vi "Begin.vi"(8 "error in":errorcluster) -> (0 "error out":errorcluster)   [LabVIEW 2018]
doc: "Called before other user functions, this VI is expected to open initial I/O refnums, load in file data, and do all program initialization. Notice that the <B>error out</B> terminal is simply used for data flow. Wiring it to other structures or subVIs ensures that this VI runs first."
uses:
  <vilib>/Rock Robotics/WPI/DriverStation/WPI_DriverStationRobotMode2.ctl
  <vilib>/Rock Robotics/WPI/Joystick/WPI_JoystickDeviceEnum.ctl
  <vilib>/Rock Robotics/WPI/ThirdParty/Phoenix-LabVIEW/Motor Controller/Controls/CTRE_Phoenix_MotorControl_ControlMode.ctl
  <vilib>/Rock Robotics/SystemInterfaces/AI/FPGA_AIChannel.ctl
  Robot Global Data.vi
  <vilib>/Rock Robotics/Network Tables/NT Write String Array.vi
panel:
  in  "Do Encoder Reset":bool
  in  "timeoutMs":u32=100
  in  "Back Right Zero":dbl=150.0
  in  "Back Left Zero":dbl=3340.0
  in  "Front Right Zero":dbl=3534.0
  in  "Front Left Zero":dbl=180.0
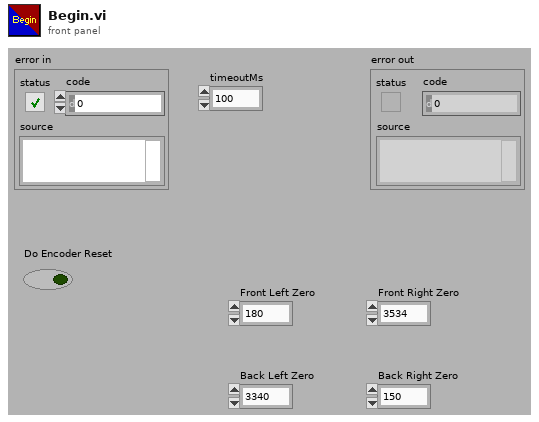
[diagram p1: front panel]
types:
  T1 = typedef "CTRE_Phoenix_MotorControl_ControlMode.ctl" = u16
  T2 = typedef "FPGA_AIChannel.ctl" = enum8{"AI 0", "AI 1", "AI 2", "AI 3", "AI MXP 0", "AI MXP 1", "AI MXP 2", "AI MXP 3", "Invalid"}
  T3 = typedef "WPI_JoystickDeviceEnum.ctl" = enum16{"USB 0", "USB 1", "USB 2", "USB 3", "USB 4", "USB 5"}
  T4 = typedef "WPI_DriverStationRobotMode2.ctl" = enum16{"Autonomous Disabled", "Autonomous Enabled", "Teleop Disabled", "Teleop Enabled", "Disconnected", "Finish", "Test Disabled", "Test Enabled", "Emergency Stopped"}
  T5 = typedef "WPI_MotorControlDeviceRef.ctl" = cluster{"DeviceStatus":errorcluster, "Type":T6, "PWM":cluster{"PWM Channel":T7, "DeadBand":T8}, "CAN":cluster{"Device Number":u8, "SetOutput VI Ref":variant, "GetOutput VI Ref":variant, "Enable VI Ref":variant, "Disable VI Ref":variant, "Data":variant}, "Invert":bool, "DIO PWM":cluster{"PWM \"Enable\" Channel":T7, "DIOChannel":T9, "PWM Rate":dbl}}
  T6 = typedef "WPI_MotorControlType.ctl" = enum16{"PWM", "CAN", "DIO PWM"}
  T7 = typedef "FPGA_DIOPWMChannel.ctl" = enum8{"PWM 0", "PWM 1", "PWM 2", "PWM 3", "PWM 4", "PWM 5", "PWM 6", "PWM 7", "PWM 8", "PWM 9", "PWM MXP 0", "PWM MXP 1", "PWM MXP 2", "PWM MXP 3", "PWM MXP 4", "PWM MXP 5", "PWM MXP 6", "PWM MXP 7", "PWM MXP 8", "PWM MXP 9", "Invalid"}
  T8 = typedef "WPI_PWMDeadband.ctl" = cluster{"Name":string, "maxPositivePwm":i32, "minPositivePwm":i32, "centerPwm":i32, "maxNegativePwm":i32, "minNegativePwm":i32, "angularRange":u16}
  T9 = typedef "FPGA_DIOChannel.ctl" = enum8{"DIO 0", "DIO 1", "DIO 2", "DIO 3", "DIO 4", "DIO 5", "DIO 6", "DIO 7", "DIO 8", "DIO 9", "DIO MXP 0", "DIO MXP 1", "DIO MXP 2", "DIO MXP 3", "DIO MXP 4", "DIO MXP 5", "DIO MXP 6", "DIO MXP 7", "DIO MXP 8", "DIO MXP 9", "DIO MXP 10", "DIO MXP 11", "DIO MXP 12", "DIO MXP 13", "DIO MXP 14", "DIO MXP 15", "SPI Port CS1", "SPI Port CS2", "SPI Port CS3", "SPI Port MISO", "SPI Port MOSI", "Invalid"}
  T10 = typedef "WPI_JoystickDevRef.ctl" = cluster{"Device":T3}
  T11 = typedef "WPI_AnalogChannelDevRef.ctl" = cluster{"DevStatus":errorcluster, "Analog Channel":T2}
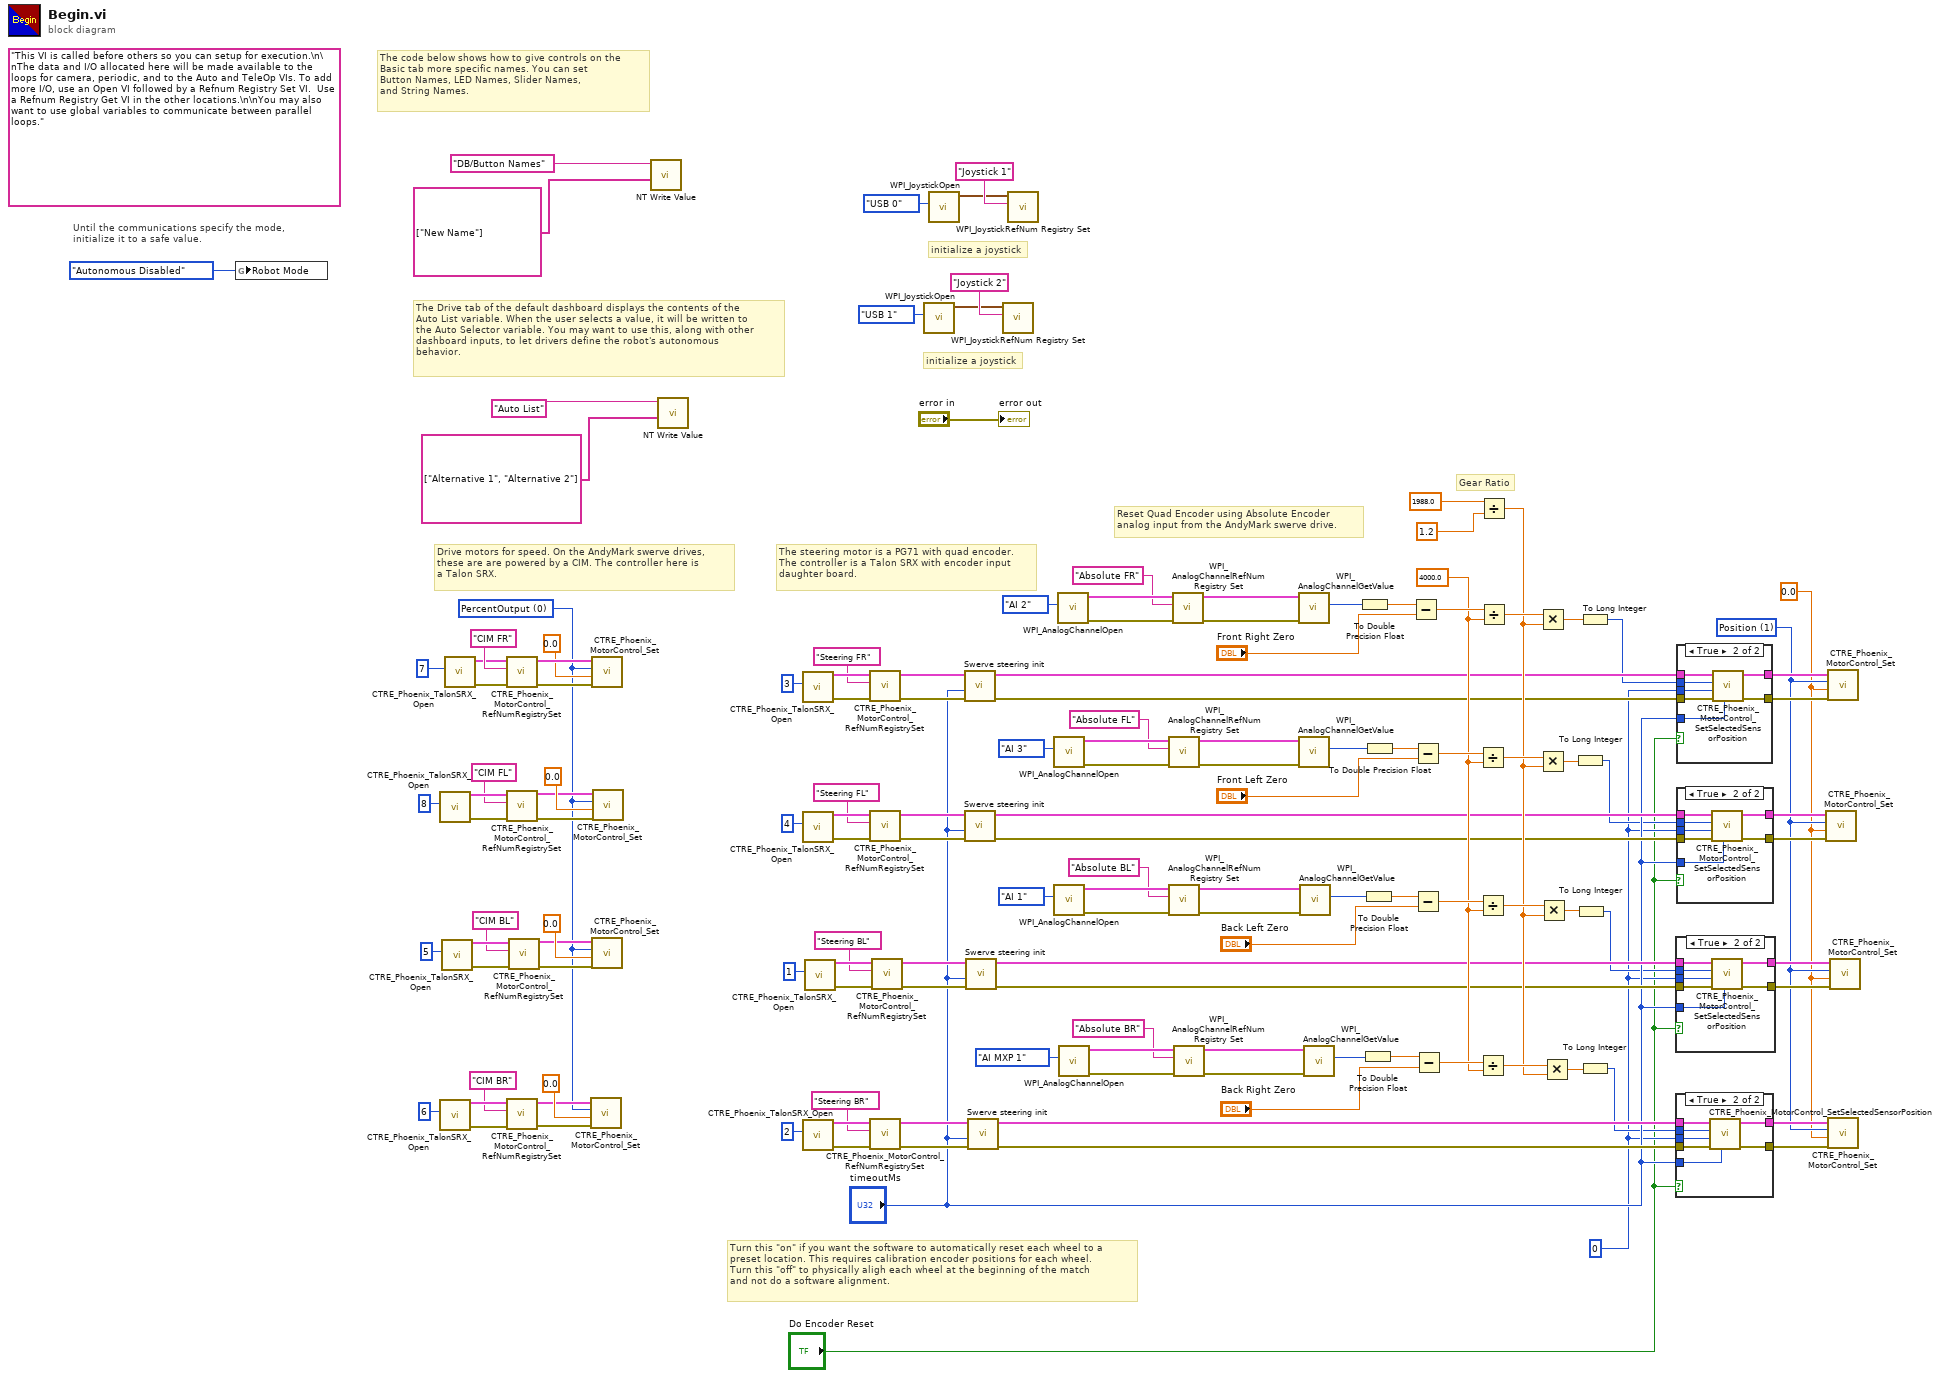
[diagram p0: block diagram]
diagram:
  w10 = 0.0 ("Output")
  w11 = T1 1 items=["PercentOutput"=0, "Position"=1, "Velocity"=2, "Current"=3, "Follower"=5, "MotionProfile"=6, "MotionMagic"=7, "MotionProfileArc"=10, "Disabled"=15] ("Control Mode")
  w20 = u32 0 ("pidLoopIdx")
  w44 = 4000.0 ("x")
  w102 = T1 0 items=["PercentOutput"=0, "Position"=1, "Velocity"=2, "Current"=3, "Follower"=5, "MotionProfile"=6, "MotionMagic"=7, "MotionProfileArc"=10, "Disabled"=15] ("Control Mode")
  (unwired) "This VI is called before others so you can setup for execution.\n\nThe data and I/O allocated here will be made available to the loops for camera, periodic, and to the Auto and TeleOp VIs. To add more I/O, use an Open VI followed by a Refnum Registry Set VI.  Use a Refnum Registry Get VI in the other locations.\n\nYou may also want to use global variables to communicate between parallel loops."
  # "The steering motor is a PG71 with quad encoder.\nThe controller is a Talon SRX with encoder input\ndaughter board."
  # "Drive motors for speed. On the AndyMark swerve drives,\nthese are are powered by a CIM. The controller here is\na Talon SRX."
  # "Turn this \"on\" if you want the software to automatically reset each wheel to a\npreset location. This requires calibration encoder positions for each wheel.\nTurn this \"off\" to physically aligh each wheel at the beginning of the match\nand not do a software alignment."
  # "Gear Ratio"
  # "Reset Quad Encoder using Absolute Encoder\nanalog input from the AndyMark swerve drive."
  # "initialize a joystick"
  # "The Drive tab of the default dashboard displays the contents of the\nAuto List variable. When the user selects a value, it will be written to\nthe Auto Selector variable. You may want to use this, along with other\ndashboard inputs, to let drivers define the robot's autonomous\nbehavior."
  # "The code below shows how to give controls on the\nBasic tab more specific names. You can set\nButton Names, LED Names, Slider Names,\nand String Names."
  # "initialize a joystick"
  # "Until the communications specify the mode,\ninitialize it to a safe value."
  n1 = global write "Robot Global Data.vi" "Robot Mode"(WPI_DriverStationRobotMode2."Autonomous Disabled" ("Robot Mode")) -> ()
  n2 = call <vilib>:"CTRE_Phoenix_TalonSRX_Open.vi"("Device Number"=u8 8) -> ("error out"=w128:errorcluster, "CAN Talon SRX Ref"=w129:T5)  [unwired: 9 in]
  n3 = call <vilib>:"CTRE_Phoenix_TalonSRX_Open.vi"("Device Number"=u8 6) -> ("error out"=w122:errorcluster, "CAN Talon SRX Ref"=w123:T5)  [unwired: 9 in]
  n4 = call <vilib>:"CTRE_Phoenix_TalonSRX_Open.vi"("Device Number"=u8 5) -> ("error out"=w125:errorcluster, "CAN Talon SRX Ref"=w126:T5)  [unwired: 9 in]
  n5 = call <vilib>:"CTRE_Phoenix_TalonSRX_Open.vi"("Device Number"=u8 7) -> ("error out"=w109:errorcluster, "CAN Talon SRX Ref"=w110:T5)  [unwired: 9 in]
  n6 = call <vilib>:"CTRE_Phoenix_MotorControl_RefNumRegistrySet.vi"("error in (no error)"=w109, "refnum name"="CIM FR", "PhoenixMotorControlDevRef"=w110) -> ("error out"=w120:errorcluster, "PhoenixMotorControlDevRef"=w119:T5)  [unwired: 7 in]
  n7 = call <vilib>:"CTRE_Phoenix_MotorControl_RefNumRegistrySet.vi"("error in (no error)"=w128, "refnum name"="CIM FL", "PhoenixMotorControlDevRef"=w129) -> ("error out"=w107:errorcluster, "PhoenixMotorControlDevRef"=w108:T5)  [unwired: 7 in]
  n8 = call <vilib>:"CTRE_Phoenix_MotorControl_RefNumRegistrySet.vi"("error in (no error)"=w122, "refnum name"="CIM BR", "PhoenixMotorControlDevRef"=w123) -> ("error out"=w113:errorcluster, "PhoenixMotorControlDevRef"=w114:T5)  [unwired: 7 in]
  n9 = call <vilib>:"CTRE_Phoenix_MotorControl_RefNumRegistrySet.vi"("error in (no error)"=w125, "refnum name"="CIM BL", "PhoenixMotorControlDevRef"=w126) -> ("error out"=w111:errorcluster, "PhoenixMotorControlDevRef"=w112:T5)  [unwired: 7 in]
  n10 = call <vilib>:"CTRE_Phoenix_MotorControl_Set.vi"("error in (no error)"=w113, "Output"=0.0, "Control Mode"=w102, "PhoenixMotorControlDevRef"=w114) -> ()  [unwired: 6 in, 2 out]
  n11 = call <vilib>:"CTRE_Phoenix_MotorControl_Set.vi"("error in (no error)"=w120, "Output"=0.0, "Control Mode"=w102, "PhoenixMotorControlDevRef"=w119) -> ()  [unwired: 6 in, 2 out]
  n12 = call <vilib>:"CTRE_Phoenix_MotorControl_Set.vi"("error in (no error)"=w111, "Output"=0.0, "Control Mode"=w102, "PhoenixMotorControlDevRef"=w112) -> ()  [unwired: 6 in, 2 out]
  n13 = call <vilib>:"CTRE_Phoenix_MotorControl_Set.vi"("error in (no error)"=w107, "Output"=0.0, "Control Mode"=w102, "PhoenixMotorControlDevRef"=w108) -> ()  [unwired: 6 in, 2 out]
  n14 = call-poly <vilib>:"NT Write Value.vi"("String Array"=string[] ["New Name"], "Name"="DB/Button Names") -> ()  [unwired: 9 in, 1 out]
  n15 = call-poly <vilib>:"NT Write Value.vi"("String Array"=string[] ["Alternative 1", "Alternative 2"], "Name"="Auto List") -> ()  [unwired: 9 in, 1 out]
  n16 = call <vilib>:"CTRE_Phoenix_TalonSRX_Open.vi"("Device Number"=u8 3) -> ("error out"=w100:errorcluster, "CAN Talon SRX Ref"=w101:T5)  [unwired: 9 in]
  n17 = call <vilib>:"CTRE_Phoenix_TalonSRX_Open.vi"("Device Number"=u8 4) -> ("error out"=w97:errorcluster, "CAN Talon SRX Ref"=w98:T5)  [unwired: 9 in]
  n18 = call <vilib>:"CTRE_Phoenix_TalonSRX_Open.vi"("Device Number"=u8 2) -> ("error out"=w91:errorcluster, "CAN Talon SRX Ref"=w92:T5)  [unwired: 9 in]
  n19 = call <vilib>:"CTRE_Phoenix_TalonSRX_Open.vi"("Device Number"=u8 1) -> ("error out"=w94:errorcluster, "CAN Talon SRX Ref"=w95:T5)  [unwired: 9 in]
  n20 = call <vilib>:"CTRE_Phoenix_MotorControl_RefNumRegistrySet.vi"("error in (no error)"=w100, "refnum name"="Steering FR", "PhoenixMotorControlDevRef"=w101) -> ("error out"=w84:errorcluster, "PhoenixMotorControlDevRef"=w85:T5)  [unwired: 7 in]
  n21 = call <vilib>:"CTRE_Phoenix_MotorControl_RefNumRegistrySet.vi"("error in (no error)"=w97, "refnum name"="Steering FL", "PhoenixMotorControlDevRef"=w98) -> ("error out"=w82:errorcluster, "PhoenixMotorControlDevRef"=w83:T5)  [unwired: 7 in]
  n22 = call <vilib>:"CTRE_Phoenix_MotorControl_RefNumRegistrySet.vi"("error in (no error)"=w91, "refnum name"="Steering BR", "PhoenixMotorControlDevRef"=w92) -> ("error out"=w78:errorcluster, "PhoenixMotorControlDevRef"=w79:T5)  [unwired: 7 in]
  n23 = call <vilib>:"CTRE_Phoenix_MotorControl_RefNumRegistrySet.vi"("error in (no error)"=w94, "refnum name"="Steering BL", "PhoenixMotorControlDevRef"=w95) -> ("error out"=w80:errorcluster, "PhoenixMotorControlDevRef"=w81:T5)  [unwired: 7 in]
  n24 = call <vilib>:"WPI_JoystickOpen.vi"("JoystickDevice"=WPI_JoystickDeviceEnum."USB 1") -> ("JoystickDevRef"=w132:T10)  [unwired: 10 in]
  n25 = call <vilib>:"WPI_JoystickOpen.vi"("JoystickDevice"=WPI_JoystickDeviceEnum."USB 0") -> ("JoystickDevRef"=w140:T10)  [unwired: 10 in]
  n26 = call "Swerve steering init.vi"("error in (no error)"=w84, "timeoutMs"="timeoutMs", "PhoenixMotorControlDevRef In"=w85) -> ("error out"=w37:errorcluster, "PhoenixMotorControlDevRef Out"=w36:T5)  [unwired: 7 in]
  n27 = call "Swerve steering init.vi"("error in (no error)"=w82, "timeoutMs"="timeoutMs", "PhoenixMotorControlDevRef In"=w83) -> ("error out"=w34:errorcluster, "PhoenixMotorControlDevRef Out"=w35:T5)  [unwired: 7 in]
  n28 = call "Swerve steering init.vi"("error in (no error)"=w80, "timeoutMs"="timeoutMs", "PhoenixMotorControlDevRef In"=w81) -> ("error out"=w32:errorcluster, "PhoenixMotorControlDevRef Out"=w33:T5)  [unwired: 7 in]
  n29 = call "Swerve steering init.vi"("error in (no error)"=w78, "timeoutMs"="timeoutMs", "PhoenixMotorControlDevRef In"=w79) -> ("error out"=w30:errorcluster, "PhoenixMotorControlDevRef Out"=w31:T5)  [unwired: 7 in]
  n30 = call <vilib>:"WPI_JoystickRefNum Registry Set.vi"("refnum name"="Joystick 2", "JoystickDevRef"=w132) -> ()  [unwired: 8 in, 2 out]
  n31 = call <vilib>:"WPI_JoystickRefNum Registry Set.vi"("refnum name"="Joystick 1", "JoystickDevRef"=w140) -> ()  [unwired: 8 in, 2 out]
  n32 = call <vilib>:"WPI_AnalogChannelOpen.vi"("Analog Channel"=FPGA_AIChannel."AI 3") -> ("error out"=w74:errorcluster, "AIDeviceRef"=w73:T11)  [unwired: 9 in]
  n33 = call <vilib>:"WPI_AnalogChannelOpen.vi"("Analog Channel"=FPGA_AIChannel."AI 1") -> ("error out"=w71:errorcluster, "AIDeviceRef"=w70:T11)  [unwired: 9 in]
  n34 = call <vilib>:"WPI_AnalogChannelOpen.vi"("Analog Channel"=FPGA_AIChannel."AI 2") -> ("error out"=w77:errorcluster, "AIDeviceRef"=w76:T11)  [unwired: 9 in]
  n35 = call <vilib>:"WPI_AnalogChannelOpen.vi"("Analog Channel"=FPGA_AIChannel."AI MXP 1") -> ("error out"=w68:errorcluster, "AIDeviceRef"=w67:T11)  [unwired: 9 in]
  n36 = call <vilib>:"WPI_AnalogChannelRefNum Registry Set.vi"("error in (no error)"=w74, "refnum name"="Absolute FL", "AIDeviceRef"=w73) -> ("error out"=w54:errorcluster, "AIDeviceRef"=w55:T11)  [unwired: 7 in]
  n37 = call <vilib>:"WPI_AnalogChannelRefNum Registry Set.vi"("error in (no error)"=w71, "refnum name"="Absolute BL", "AIDeviceRef"=w70) -> ("error out"=w57:errorcluster, "AIDeviceRef"=w56:T11)  [unwired: 7 in]
  n38 = call <vilib>:"WPI_AnalogChannelRefNum Registry Set.vi"("error in (no error)"=w77, "refnum name"="Absolute FR", "AIDeviceRef"=w76) -> ("error out"=w60:errorcluster, "AIDeviceRef"=w61:T11)  [unwired: 7 in]
  n39 = call <vilib>:"WPI_AnalogChannelRefNum Registry Set.vi"("error in (no error)"=w68, "refnum name"="Absolute BR", "AIDeviceRef"=w67) -> ("error out"=w58:errorcluster, "AIDeviceRef"=w59:T11)  [unwired: 7 in]
  n40 = call <vilib>:"WPI_AnalogChannelGetValue.vi"("error in (no error)"=w60, "AIDeviceRef"=w61) -> ("Value"=w7:i16)  [unwired: 7 in, 2 out]
  n41 = call <vilib>:"WPI_AnalogChannelGetValue.vi"("error in (no error)"=w54, "AIDeviceRef"=w55) -> ("Value"=w5:i16)  [unwired: 7 in, 2 out]
  n42 = call <vilib>:"WPI_AnalogChannelGetValue.vi"("error in (no error)"=w57, "AIDeviceRef"=w56) -> ("Value"=w3:i16)  [unwired: 7 in, 2 out]
  n43 = call <vilib>:"WPI_AnalogChannelGetValue.vi"("error in (no error)"=w58, "AIDeviceRef"=w59) -> ("Value"=w9:i16)  [unwired: 7 in, 2 out]
  n44 = To Double Precision Float(number=w7) -> (double precision float=w6:dbl)
  n45 = To Double Precision Float(number=w9) -> (double precision float=w8:dbl)
  n46 = To Double Precision Float(number=w3) -> (double precision float=w2:dbl)
  n47 = To Double Precision Float(number=w5) -> (double precision float=w4:dbl)
  n48 = Subtract(x=w6, y="Front Right Zero") -> (x-y=w48:dbl)
  n49 = Subtract(x=w4, y="Front Left Zero") -> (x-y=w47:dbl)
  n50 = Subtract(x=w2, y="Back Left Zero") -> (x-y=w46:dbl)
  n51 = Subtract(x=w8, y="Back Right Zero") -> (x-y=w45:dbl)
  n52 = Divide(x=w47, y=w44) -> (x/y=w39:dbl)
  n53 = Divide(x=w46, y=w44) -> (x/y=w40:dbl)
  n54 = Divide(x=w45, y=w44) -> (x/y=w41:dbl)
  n55 = Divide(x=1988.0 ("y"), y=1.2) -> (x/y=w38:dbl)
  n56 = Divide(x=w48, y=w44) -> (x/y=w42:dbl)
  n57 = Multiply(x=w42, y=w38) -> (x*y=w28:dbl)
  n58 = Multiply(x=w39, y=w38) -> (x*y=w26:dbl)
  n59 = Multiply(x=w40, y=w38) -> (x*y=w25:dbl)
  n60 = Multiply(x=w41, y=w38) -> (x*y=w24:dbl)
  n61 = To Long Integer(number=w26) -> (32bit integer=w23:i32)
  n62 = To Long Integer(number=w25) -> (32bit integer=w22:i32)
  n63 = To Long Integer(number=w28) -> (32bit integer=w27:i32)
  n64 = To Long Integer(number=w24) -> (32bit integer=w21:i32)
  n65 = case shown="True" "Do Encoder Reset" {
    tunnel: w33 -> [w144 w151]
    tunnel: w32 -> [w143 w150]
    tunnel: "timeoutMs" -> [_ w149]
    tunnel: w22 -> [_ w148]
    tunnel: w20 -> [_ w147]
    tunnel: [w143 w146] -> w15
    tunnel: [w144 w145] -> w14
    frame False {
    }
    frame True {
      n66 = call <vilib>:"CTRE_Phoenix_MotorControl_SetSelectedSensorPosition.vi"("timeoutMs"=w149, "error in (no error)"=w150, "pidLoopIdx"=w147, "New Sensor Position"=w148, "PhoenixMotorControlDevRef"=w151) -> ("error out"=w146:errorcluster, "PhoenixMotorControlDevRef"=w145:T5)  [unwired: 5 in]
    }
  }
  n67 = case shown="True" "Do Encoder Reset" {
    tunnel: w31 -> [w153 w160]
    tunnel: w30 -> [w152 w159]
    tunnel: "timeoutMs" -> [_ w158]
    tunnel: w21 -> [_ w157]
    tunnel: w20 -> [_ w156]
    tunnel: [w153 w155] -> w17
    tunnel: [w152 w154] -> w16
    frame False {
    }
    frame True {
      n68 = call <vilib>:"CTRE_Phoenix_MotorControl_SetSelectedSensorPosition.vi"("timeoutMs"=w158, "error in (no error)"=w159, "pidLoopIdx"=w156, "New Sensor Position"=w157, "PhoenixMotorControlDevRef"=w160) -> ("error out"=w154:errorcluster, "PhoenixMotorControlDevRef"=w155:T5)  [unwired: 5 in]
    }
  }
  n69 = case shown="True" "Do Encoder Reset" {
    tunnel: w37 -> [w161 w169]
    tunnel: w36 -> [w162 w168]
    tunnel: "timeoutMs" -> [_ w167]
    tunnel: w27 -> [_ w166]
    tunnel: w20 -> [_ w165]
    tunnel: [w161 w164] -> w19
    tunnel: [w162 w163] -> w18
    frame False {
    }
    frame True {
      n70 = call <vilib>:"CTRE_Phoenix_MotorControl_SetSelectedSensorPosition.vi"("timeoutMs"=w167, "error in (no error)"=w169, "pidLoopIdx"=w165, "New Sensor Position"=w166, "PhoenixMotorControlDevRef"=w168) -> ("error out"=w164:errorcluster, "PhoenixMotorControlDevRef"=w163:T5)  [unwired: 5 in]
    }
  }
  n71 = case shown="True" "Do Encoder Reset" {
    tunnel: w35 -> [w171 w178]
    tunnel: w34 -> [w170 w177]
    tunnel: "timeoutMs" -> [_ w176]
    tunnel: w23 -> [_ w175]
    tunnel: w20 -> [_ w174]
    tunnel: [w170 w173] -> w13
    tunnel: [w171 w172] -> w12
    frame False {
    }
    frame True {
      n72 = call <vilib>:"CTRE_Phoenix_MotorControl_SetSelectedSensorPosition.vi"("timeoutMs"=w176, "error in (no error)"=w177, "pidLoopIdx"=w174, "New Sensor Position"=w175, "PhoenixMotorControlDevRef"=w178) -> ("error out"=w173:errorcluster, "PhoenixMotorControlDevRef"=w172:T5)  [unwired: 5 in]
    }
  }
  n73 = call <vilib>:"CTRE_Phoenix_MotorControl_Set.vi"("error in (no error)"=w13, "Output"=w10, "Control Mode"=w11, "PhoenixMotorControlDevRef"=w12) -> ()  [unwired: 6 in, 2 out]
  n74 = call <vilib>:"CTRE_Phoenix_MotorControl_Set.vi"("error in (no error)"=w19, "Output"=w10, "Control Mode"=w11, "PhoenixMotorControlDevRef"=w18) -> ()  [unwired: 6 in, 2 out]
  n75 = call <vilib>:"CTRE_Phoenix_MotorControl_Set.vi"("error in (no error)"=w16, "Output"=w10, "Control Mode"=w11, "PhoenixMotorControlDevRef"=w17) -> ()  [unwired: 6 in, 2 out]
  n76 = call <vilib>:"CTRE_Phoenix_MotorControl_Set.vi"("error in (no error)"=w15, "Output"=w10, "Control Mode"=w11, "PhoenixMotorControlDevRef"=w14) -> ()  [unwired: 6 in, 2 out]
  "error out" <- "error in"
